vi "Read.vi"(6 "Append Index":i32, 8 "error in (no error)":errorcluster, 11 "Data.PG in":refnum<class "LV-Data.PGSQL.lvclass">) -> (0 "error out":errorcluster, 1 "Notes":string, 2 "Data (Dictionary)":T1[](array[typedef]), 3 "Data.PG out":refnum<class "LV-Data.PGSQL.lvclass">, 5 "Path out":path)   [LabVIEW 2019, in "LV-Data.PGSQL.lvclass"]
uses:
  LV-Data.PGSQL.lvclass
  C:/Program Files (x86)/National Instruments/LabVIEW 2019/user.lib/LevyLab/LV-Data/LV-Data/LV-Data.lvclass
  <userlib>/LevyLab/LV-Data/LV-Data/Typedefs/Dictionary--cluster.ctl
  <vilib>/JDP Science/PostgreSQL Library/Connection/PQ Connection.lvclass
  LV-Data.PGSQL.lvclass/LV-Data.PGSQL.ctl
  <userlib>/LevyLab/LV-Data/LV-Data/Typedefs/Operation--enum.ctl
  <userlib>/LevyLab/LV-Data/LV-Data/LV-Data.lvclass/LV-Data.ctl
  <vilib>/JDP Science/PostgreSQL Library/Connection/Execute Command (2D string results).vi
  <vilib>/JDP Science/PostgreSQL Library/Connection/Execute Command (Result).vi
  <vilib>/JDP Science/PostgreSQL Library/Result/Get all results as 2D strings array.vi
  <vilib>/JDP Science/PostgreSQL Library/Result/Get Column Headers.vi
  <vilib>/JDP Science/PostgreSQL Library/Result/Clear.vi
  <userlib>/LevyLab/LV-Data/LV-Data/LV-Data.lvclass
  <vilib>/JDP Science/PostgreSQL Library/Result/PQ Result.lvclass
panel:
  out "size(s)":i32[](array[numeric])
  out "Result":string[][](array[string])
  in  "command":string="SELECT * FROM test_table where my_dbl>0.99;"
  # "MNK"
  # "fsfdfsglkjjjb"
  # "SAMPLE"
  # "GUID EXPT#?"
  # "time"
  # "INST"
  # "ID#"
  # "Vsg"
  # "T"
  # "B"
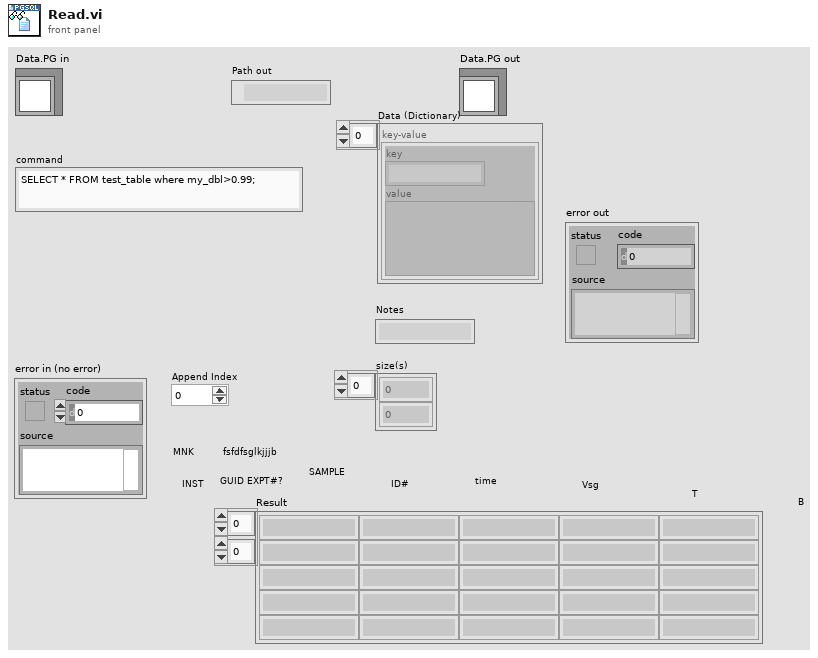
[diagram p1: front panel]
types:
  T1 = typedef "LV-Data.lvclass/Dictionary--cluster.ctl" = cluster{"key":string, "value":variant}
  T2 = typedef "LV-Data.lvclass/Operation--enum.ctl" = enum16{"Read", "Write", "Write + Append"}
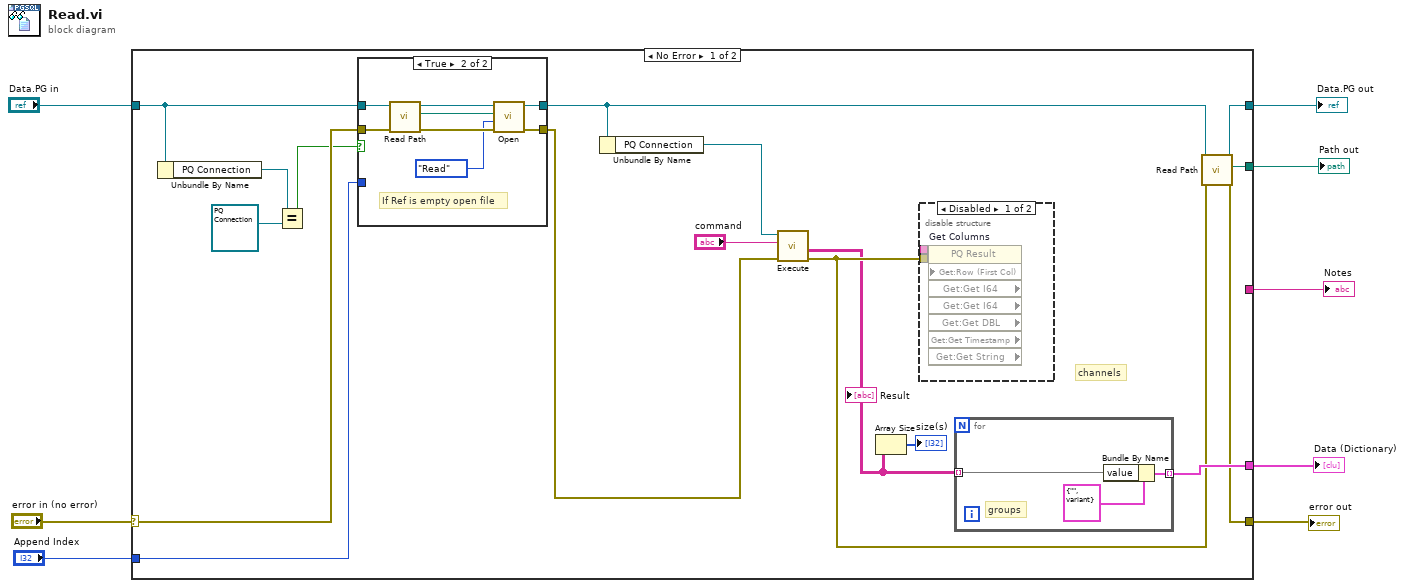
[diagram p0: block diagram]
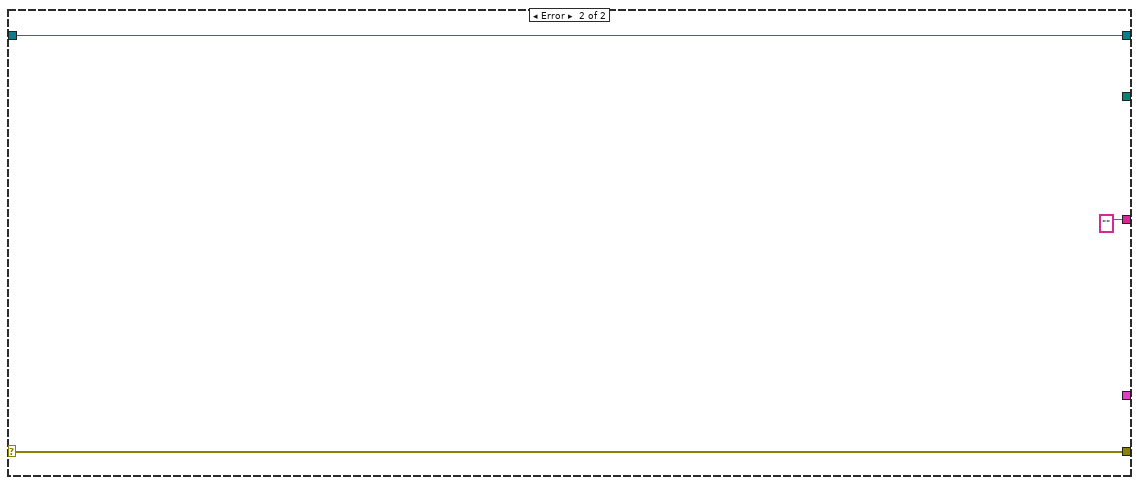
[diagram p4: hidden frame]
diagram:
  n1 = case shown="No Error" "error in (no error)" {
    selector: "error in (no error)" -> [w20 w43]
    tunnel: "Data.PG in" -> [w21 w42]
    tunnel: [w23 w42] -> w7
    tunnel: [w22 w43] -> w6
    tunnel: [w24 _] -> w5
    tunnel: "Append Index" -> [w16 _]
    tunnel: [w25 _] -> w1
    tunnel: [_ ""] -> w2
    frame No Error {
      # "channels"
      n2 = Unbundle By Name(w21) -> ("PQ Connection"=w18:refnum<class "PQ Connection.lvclass">)
      n3 = Equal?(x=w18, y=refnum<class "PQ Connection.lvclass"> refnum ("PQ Connection")) -> (x = y?=w17:bool)
      n4 = case shown="True" w17 {
        tunnel: w21 -> [w31 w36]
        tunnel: [w31 w40] -> w9
        tunnel: [w32 w38] -> w15
        tunnel: w20 -> [w32 w37]
        tunnel: w16 -> [_ _]
        frame False {
        }
        frame True {
          # "If Ref is empty open file"
          n5 = call <userlib>:"Read Path.vi"("error in (no error)"=w37, "Data Save"=w36) -> ("error out"=w39:errorcluster, "Path"=w34:path, "Data Save out"=w35:refnum<class "LV-Data.PGSQL.lvclass">)  [unwired: 7 in]
          n6 = call-dynamic "Open.vi"("error in (no error)"=w39, "Operation"=Operation--enum."Read", "Path"=w34, "Data in"=w35) -> ("error out"=w38:errorcluster, "Data out"=w40:refnum<class "LV-Data.PGSQL.lvclass">)  [unwired: 6 in]
        }
      }
      n7 = Unbundle By Name(w9) -> ("PQ Connection"=w13:refnum<class "PQ Connection.lvclass">)
      n8 = call-poly <vilib>:"Execute.vi"("error in (no error)"=w15, "SQL"="command", "PQ Connection in"=w13) -> ("error out"=w12:errorcluster, "Result"=w11:string[][])  [unwired: 4 in, 3 out]
      "Result" <- w11
      n9 = Array Size(array=w11) -> (size(s)=→"size(s)":i32[])
      n10 = disable-structure shown="Disabled" {
        disable-tunnel: _ -> [w30 _]
        disable-tunnel: w12 -> [w29 _]
        frame Disabled {
          n11 = property on="Get Columns" class="PQ Result" props=["Get:Row (First Col)", "Get:Get I64", "Get:Get I64", "Get:Get DBL", "Get:Get Timestamp", "Get:Get String"](reference=w30, error in=w29) -> ()  [unwired: 1 in, 7 out]
        }
        frame Enabled {
        }
      }
      n12 = for {
        tunnel: [w28] -> w25 mode=indexing
        tunnel: w11 -> [w26] mode=indexing
        # "groups"
        n13 = Bundle By Name(cluster=T1 {"key"="", "value"=variant} ("key-value"), "value"=w26) -> (w28:T1)
      }
      n14 = call <userlib>:"Read Path.vi"("error in (no error)"=w12, "Data Save"=w9) -> ("error out"=w22:errorcluster, "Path"=w24:path, "Data Save out"=w23:refnum<class "LV-Data.PGSQL.lvclass">)  [unwired: 7 in]
    }
    frame Error {
    }
  }
  "error out" <- w6
  "Data.PG out" <- w7
  "Path out" <- w5
  "Data (Dictionary)" <- w1
  "Notes" <- w2
